vi "CAD@AddRobot__Parameter.vi"(1 "ParamterIn":string) -> (0 "ParamterOut":string)   [LabVIEW 2020]
panel:
  in  "Model":string(combo)
  in  "RobotName":string(combo)
  in  "Confirm":bool
  # "CAD@AddRobot $Part,$Model"
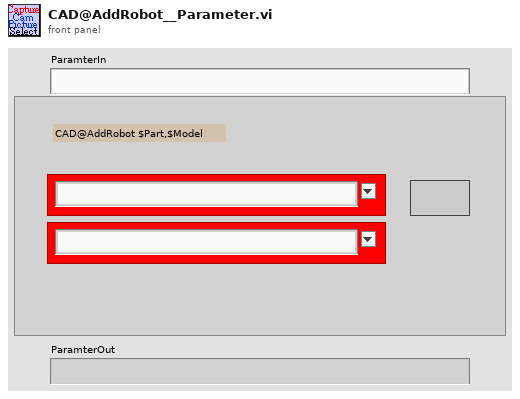
[diagram p1: front panel]
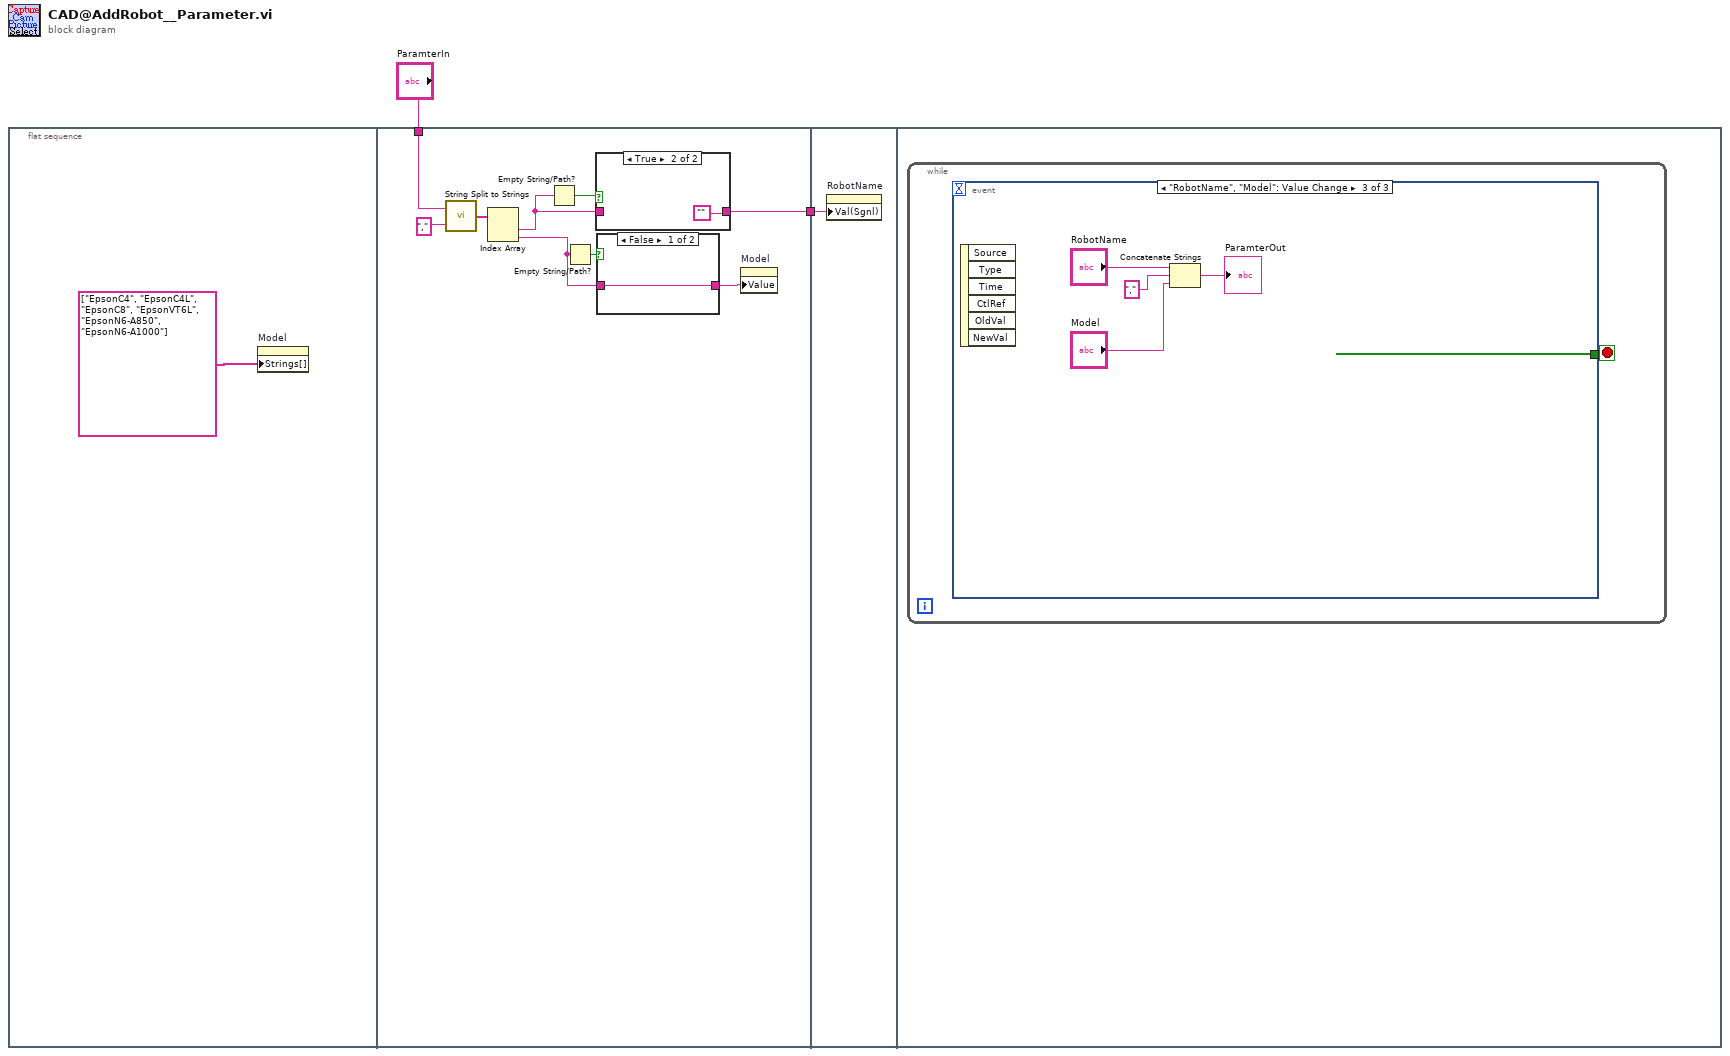
[diagram p0: block diagram]
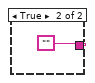
[diagram p2: hidden frame]
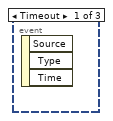
[diagram p4: hidden frame]
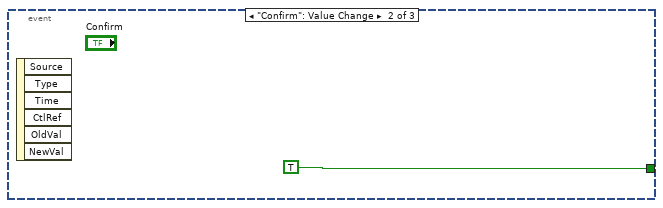
[diagram p5: hidden frame]
diagram:
  n1 = flat-sequence {
    tunnel: "ParamterIn" -> [w10]
    tunnel: [w5] -> w1
    tunnel: w1 -> [w17]
    frame #0 {
      n2 = property on="Model" class="CmbBox"("Strings[]"=string[] ["EpsonC4", "EpsonC4L", "EpsonC8", "EpsonVT6L", "EpsonN6-A850", "EpsonN6-A1000"] ("Strings []")) -> ()  [unwired: 2 in, 2 out]
    }
    frame #1 {
      n3 = call "String Split to Strings.vi"("search string/char (-)"=",", "String"=w10) -> ("Array"=w12:string[])
      n4 = Index Array(array=w12) -> (element #1=w6:string, element #2=w7:string)  [unwired: 2 in]
      n5 = Empty String/Path?(string/path=w6) -> (empty?=w9:bool)
      n6 = Empty String/Path?(string/path=w7) -> (empty?=w8:bool)
      n7 = case shown="True" w9 {
        tunnel: w6 -> [w15 _]
        tunnel: [w15 ""] -> w5
        frame False {
        }
        frame True {
        }
      }
      n8 = case shown="False" w8 {
        tunnel: [w13 ""] -> w4
        tunnel: w7 -> [w13 _]
        frame False {
        }
        frame True {
        }
      }
      n9 = property on="Model" class="CmbBox"("Value"=w4) -> ()  [unwired: 2 in, 2 out]
    }
    frame #2 {
      n10 = property on="RobotName" class="CmbBox"("Val(Sgnl)"=w17) -> ()  [unwired: 2 in, 2 out]
    }
    frame #3 {
      n11 = while {
        stop <- w18 stop-if-true
        n12 = event shown="[2] \"RobotName\", \"Model\": Value Change" {
          selector: _ -> [_ _ _]
          dyn-events: _ -> [_ _ _]
          timeout: _ -> [_ _ _]
          tunnel: [_ TRUE _] -> w18
          event Timeout {
            n13 = event-data() -> ()  [unwired: 1 in, 3 out]
          }
          event "Confirm": Value Change {
            n14 = event-data() -> ()  [unwired: 1 in, 6 out]
          }
          event "RobotName", "Model": Value Change {
            n15 = event-data() -> ()  [unwired: 1 in, 6 out]
            n16 = Concatenate Strings("RobotName", "," ("element"), "Model") -> (→"ParamterOut":string)
          }
        }
      }
    }
  }
